vi "Call Worker Drop Instance.vi"(10 "error in (no error)":errorcluster, 11 "Worker Path In":path) -> (2 "error out":errorcluster, 3 "Worker Path":path)   [LabVIEW 2022 SP3, in "FlexBlocks Support.lvlib"]
uses:
  FlexBlocks Support.lvlib
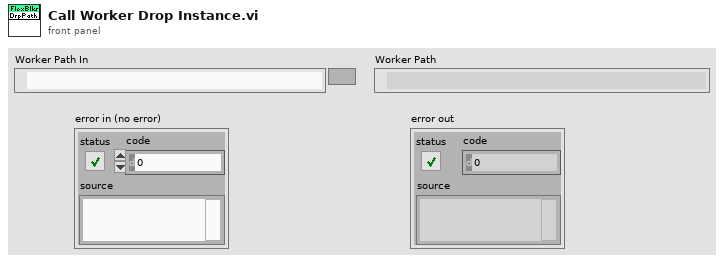
[diagram p1: front panel]
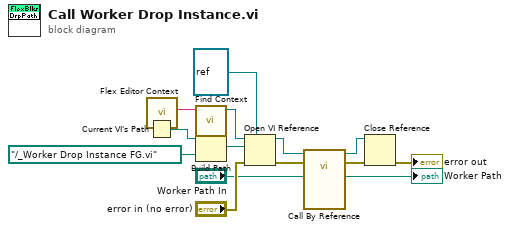
[diagram p0: block diagram]
diagram:
  n1 = call "Flex Editor Context.vi"() -> ("Flex Editor Context"=w13:string)  [unwired: 11 in]
  n2 = Current VI's Path() -> (path=w11:path)
  n3 = call "Find Context.vi"("Name"=w13) -> ("App"=w12:refnum<vi>)  [unwired: 9 in, 1 out]
  n4 = Build Path(base path=w11, name or relative path=path "../_Worker Drop Instance FG.vi") -> (appended path=w9:path)
  n5 = Open VI Reference(type specifier VI Refnum (for type only)=refnum<vi> refnum, application reference (local)=w12, vi path=w9, error in (no error)="error in (no error)") -> (vi reference=w6:refnum<vi>, error out=w7:errorcluster)  [unwired: 2 in]
  n6 = call-by-ref "?"(reference=w6, error in=w7, "Worker Path In"="Worker Path In") -> (reference out=w2:refnum<vi>, error out=w3:errorcluster, "Worker Path"=→"Worker Path":path)  [unwired: 10 in]
  n7 = Close Reference(reference=w2, error in (no error)=w3) -> (error out=→"error out":errorcluster)
